vi "ChangeMemAllocation.vi"(8 "error in (no error)":errorcluster, 11 "Astar Open List in":refnum<class "NI_Robotics_Priority Queue.lvclass">) -> (0 "error out":errorcluster, 3 "Astar Open List out":refnum<class "NI_Robotics_Priority Queue.lvclass">)   [LabVIEW 2017, in "NI_Robotics_Priority Queue.lvclass"]
uses:
  <vilib>/robotics/Navigation/shared/Priority Queue/NI_Robotics_Priority Queue.lvclass
  <vilib>/robotics/Navigation/shared/Priority Queue/NI_Robotics_Priority Queue.lvclass/NI_Robotics_Priority Queue.ctl
panel:
  in  "Desired allocation size":i32
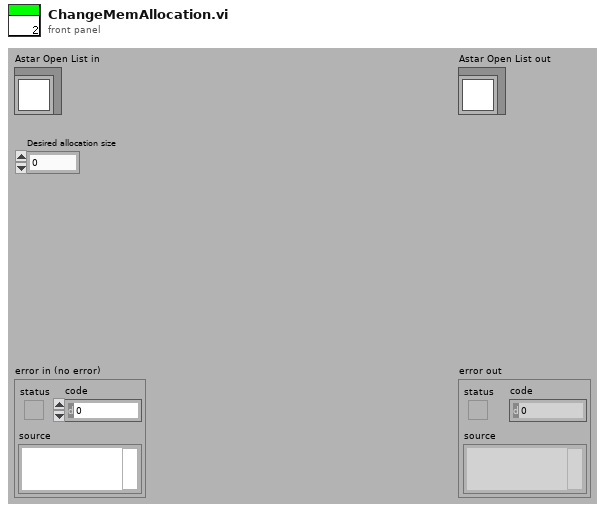
[diagram p1: front panel]
types:
  T1 = typedef "NI_Robotics_Priority Queue.lvclass/Open List Element.ctl" = cluster{"f":dbl, "g":dbl, "node Ref":refnum<data-value>}
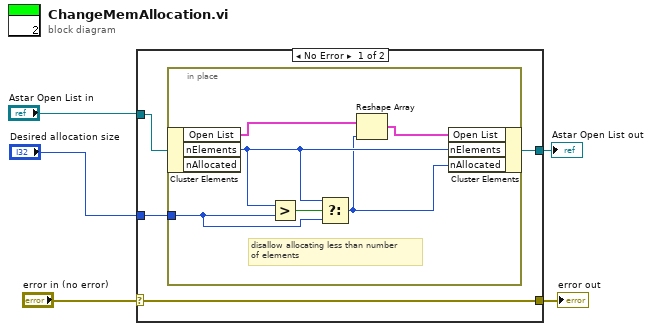
[diagram p0: block diagram]
diagram:
  n1 = case shown="No Error" "error in (no error)" {
    selector: "error in (no error)" -> [w9 w17]
    tunnel: [w9 w17] -> w4
    tunnel: "Astar Open List in" -> [w7 w16]
    tunnel: "Desired allocation size" -> [w8 _]
    tunnel: [w6 w16] -> w1
    frame No Error {
      n2 = in-place {
        in-place-border: w8 -> [w14]
        # "disallow allocating less than number\nof elements"
        n3 = in-place-cluster #1(w7) -> ("Open List"=w13:T1[], "nElements"=w11:i32)  [unwired: 1 out]
        n4 = Greater?(x=w11, y=w14) -> (0:w15:bool)
        n5 = Select(t=w11, s=w15, f=w14) -> (s? t:f=w10:i32)
        n6 = Reshape Array(w13, w10) -> (w12:T1[])
        n7 = in-place-cluster #1("Open List"=w12, "nElements"=w11, "nAllocated"=w10) -> (w6:refnum<class "NI_Robotics_Priority Queue.lvclass">)
      }
    }
    frame Error {
    }
  }
  "error out" <- w4
  "Astar Open List out" <- w1
